vi "CSVFormat.vi"(10 "TV Parameters(DataType)":T1 {"Standard" items=["80211A/G/J/P OFDM", "80211B/G DSSS", "80211G DSSSOFDM", "80211N MIMOOFDM", "80211AC MIMOOFDM"]; "OFDM Data Rate (Mbps)" items=["6", "9", "12", "18", "24", "36", "48", "54"]; "80211n PLCP Frame Format" items=["Mixed Format", "Greenfield Format"]; "FEC Coding Type" items=["BCC", "LDPC"]; "DSSS Data Rate (Mbps)" items=["1", "2", "5.5 CCK", "5.5 PBCC", "11 CCK", "11 PBCC", "22", "33"]}, 11 "WLAN TX Result":T2) -> (3 "Array":string[][](array[string]))   [LabVIEW 2012]
uses:
  Instrument Control/TV/RW/Includes/WLAN - TV - RW - INC - TV_DataType_Cluster.ctl
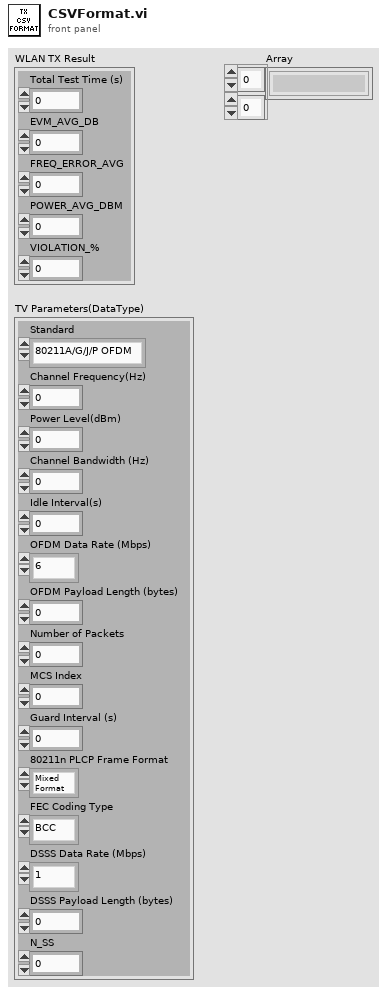
[diagram p1: front panel]
types:
  T1 = typedef "WLAN - TV - RW - INC - TV_DataType_Cluster.ctl" = cluster{"Standard":i32, "Channel Frequency(Hz)":dbl, "Power Level(dBm)":dbl, "Channel Bandwidth (Hz)":dbl, "Idle Interval(s)":dbl, "OFDM Data Rate (Mbps)":i32, "OFDM Payload Length (bytes)":i32, "Number of Packets":i32, "MCS Index":i32, "Guard Interval (s)":dbl, "80211n PLCP Frame Format":i32, "FEC Coding Type":i32, "DSSS Data Rate (Mbps)":i32, "DSSS Payload Length (bytes)":i32, "N_SS":i32}
  T2 = cluster{"Total Test Time (s)":dbl, "EVM_AVG_DB":dbl, "FREQ_ERROR_AVG":dbl, "POWER_AVG_DBM":dbl, "VIOLATION_%":dbl}
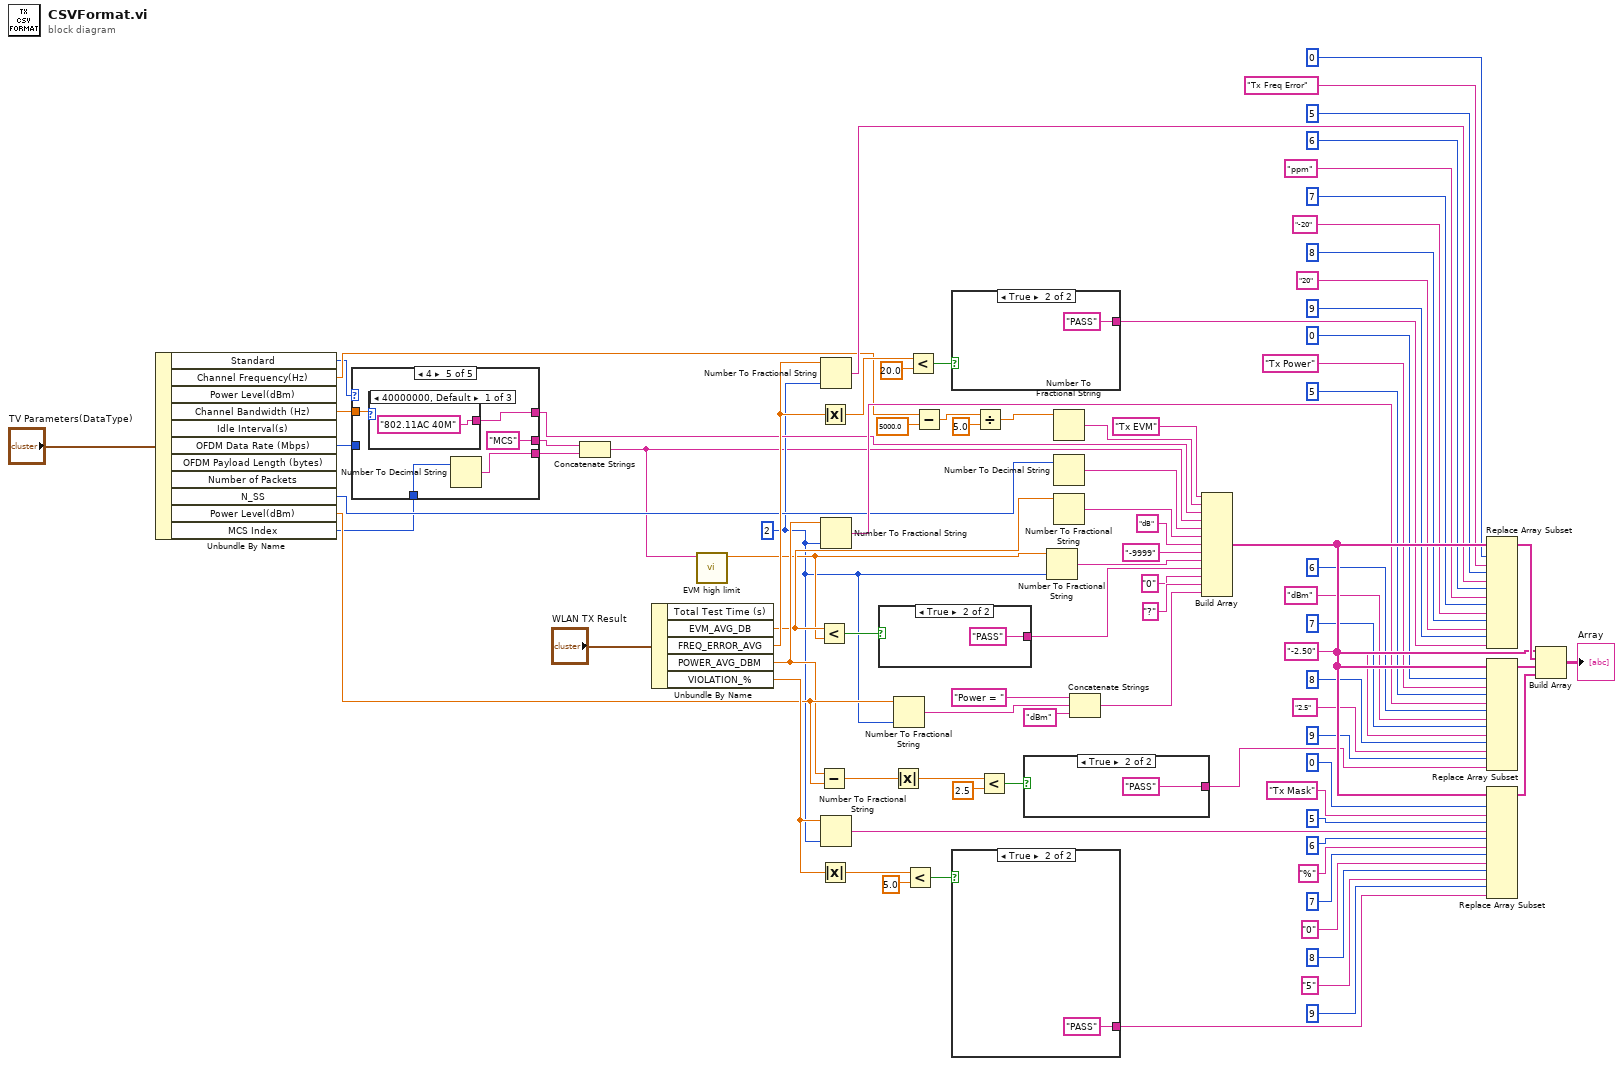
[diagram p0: block diagram]
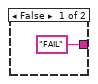
[diagram p2: hidden frame]
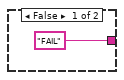
[diagram p3: hidden frame]
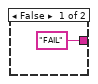
[diagram p4: hidden frame]
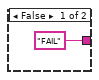
[diagram p5: hidden frame]
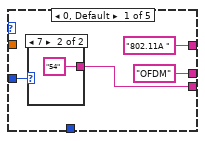
[diagram p6: hidden frame]
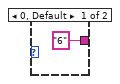
[diagram p7: hidden frame]
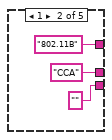
[diagram p8: hidden frame]
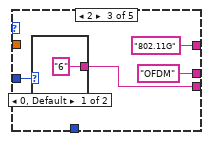
[diagram p9: hidden frame]
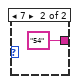
[diagram p10: hidden frame]
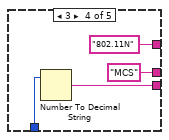
[diagram p11: hidden frame]
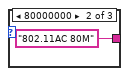
[diagram p12: hidden frame]
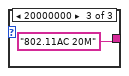
[diagram p13: hidden frame]
diagram:
  w6 = i16 2 ("width (-)")
  n1 = Unbundle By Name("TV Parameters(DataType)") -> ("Standard"=w10:i32, "Channel Frequency(Hz)"=w16:dbl, "Channel Bandwidth (Hz)"=w1:dbl, "OFDM Data Rate (Mbps)"=w5:i32, "N_SS"=w13:i32, "Power Level(dBm)"=w64:dbl, "MCS Index"=w2:i32)  [unwired: 4 out]
  n2 = case shown="4" w10 {
    tunnel: ["802.11A " "802.11B" "802.11G" "802.11N" w109] -> w11
    tunnel: ["OFDM" "CCA" "OFDM" "MCS" "MCS"] -> w12
    tunnel: w5 -> [w91 _ w99 _ _]
    tunnel: [w90 "" w100 w106 w112] -> w4
    tunnel: w2 -> [_ _ _ w105 w111]
    tunnel: w1 -> [_ _ _ _ w110]
    frame 0, Default {
      n3 = case shown="7" w91 {
        tunnel: ["6" "54"] -> w90
        frame 0, Default {
        }
        frame 7 {
        }
      }
    }
    frame 1 {
    }
    frame 2 {
      n4 = case shown="0, Default" w99 {
        tunnel: ["6" "54"] -> w100
        frame 0, Default {
        }
        frame 7 {
        }
      }
    }
    frame 3 {
      n5 = Number To Decimal String(number=w105) -> (decimal integer string=w106:string)  [unwired: 1 in]
    }
    frame 4 {
      n6 = case shown="40000000, Default" w110 {
        tunnel: ["802.11AC 40M" "802.11AC 80M" "802.11AC 20M"] -> w109
        frame 40000000, Default {
        }
        frame 80000000 {
        }
        frame 20000000 {
        }
      }
      n7 = Number To Decimal String(number=w111) -> (decimal integer string=w112:string)  [unwired: 1 in]
    }
  }
  n8 = Concatenate Strings(w12, w4) -> (w3:string)
  n9 = Unbundle By Name("WLAN TX Result") -> ("EVM_AVG_DB"=w27:dbl, "FREQ_ERROR_AVG"=w45:dbl, "POWER_AVG_DBM"=w62:dbl, "VIOLATION_%"=w83:dbl)  [unwired: 1 out]
  n10 = call "EVM high limit.vi"("MCS Index"=w3) -> ("EVM High Limit"=w26:dbl)  [unwired: 10 in]
  n11 = Less?(x=w27, y=w26) -> (x < y?=w25:bool)
  n12 = Subtract(x=w62, y=w64) -> (x-y=w59:dbl)
  n13 = Absolute Value(x=w45) -> (abs(x)=w42:dbl)
  n14 = Absolute Value(x=w83) -> (abs(x)=w82:dbl)
  n15 = Number To Fractional String(number=w45, precision (6)=w6) -> (F-format string=w34:string)  [unwired: 2 in]
  n16 = Number To Fractional String(number=w62, precision (6)=w6) -> (F-format string=w63:string)  [unwired: 2 in]
  n17 = Number To Fractional String(number=w83, precision (6)=w6) -> (F-format string=w79:string)  [unwired: 2 in]
  n18 = case shown="True" w25 {
    tunnel: ["FAIL" ("string") "PASS" ("string")] -> w28
    frame False {
    }
    frame True {
    }
  }
  n19 = Absolute Value(x=w59) -> (abs(x)=w57:dbl)
  n20 = Number To Fractional String(number=w64, precision (6)=w6) -> (F-format string=w66:string)  [unwired: 2 in]
  n21 = Less?(x=w82, y=5.0 ("upper limit")) -> (x < y?=w80:bool)
  n22 = Less?(x=w42, y=20.0) -> (x < y?=w44:bool)
  n23 = Subtract(x=w16, y=5000.0) -> (x-y=w18:dbl)
  n24 = case shown="True" w44 {
    tunnel: ["FAIL" ("string") "PASS" ("string")] -> w46
    frame False {
    }
    frame True {
    }
  }
  n25 = case shown="True" w80 {
    tunnel: ["FAIL" ("string") "PASS" ("string")] -> w84
    frame False {
    }
    frame True {
    }
  }
  n26 = Divide(x=w18, y=5.0) -> (x/y=w20:dbl)
  n27 = Less?(x=w57, y=2.5 ("upper limit")) -> (x < y?=w60:bool)
  n28 = case shown="True" w60 {
    tunnel: ["FAIL" ("string") "PASS" ("string")] -> w61
    frame False {
    }
    frame True {
    }
  }
  n29 = Number To Fractional String(number=w26, precision (6)=w6) -> (F-format string=w24:string)  [unwired: 2 in]
  n30 = Number To Fractional String(number=w20) -> (F-format string=w21:string)  [unwired: 3 in]
  n31 = Number To Decimal String(number=w13) -> (decimal integer string=w14:string)  [unwired: 1 in]
  n32 = Number To Fractional String(number=w27) -> (F-format string=w15:string)  [unwired: 3 in]
  n33 = Concatenate Strings("Power = ", w66, "dBm" ("string")) -> (w68:string)
  n34 = Build Array("Tx EVM", w21, w11, w3, w14, w15, "dB" ("element"), "-9999" ("element"), w24, w28, "0" ("element"), "?" ("element"), w68) -> (w85:string[])
  n35 = Replace Array Subset(array=w85, new element #1="Tx Freq Error" ("new element/subarray"), index #1=0 ("index"), new element #2=w34, index #2=5 ("index"), new element #3="ppm" ("new element/subarray"), index #3=6 ("index"), new element #4="-20" ("new element/subarray"), index #4=7 ("index"), new element #5="20" ("new element/subarray"), index #5=8 ("index"), new element #6=w46, index #6=9 ("index")) -> (w86:string[])
  n36 = Replace Array Subset(array=w85, new element #1="Tx Power" ("new element/subarray"), index #1=0 ("index"), new element #2=w63, index #2=5 ("index"), new element #3="dBm" ("new element/subarray"), index #3=6 ("index"), new element #4="-2.50" ("new element/subarray"), index #4=7 ("index"), new element #5="2.5" ("new element/subarray"), index #5=8 ("index"), new element #6=w61, index #6=9 ("index")) -> (w87:string[])
  n37 = Replace Array Subset(array=w85, new element #1="Tx Mask" ("new element/subarray"), index #1=0 ("index"), new element #2=w79, index #2=5 ("index"), new element #3="%" ("new element/subarray"), index #3=6 ("index"), new element #4="0" ("new element/subarray"), index #4=7 ("index"), new element #5="5" ("new element/subarray"), index #5=8 ("index"), new element #6=w84, index #6=9 ("index")) -> (w88:string[])
  n38 = Build Array(w85, w86, w87, w88) -> (→"Array":string[][])
